vi "X509_store_get_size.vi"(8 "error in (no error)":errorcluster, 11 "SSL-Context in":refnum<class "SSL-Context.lvclass">) -> (0 "error out":errorcluster, 2 "Size of X509 Store":i32, 3 "SSL-Context out":refnum<class "SSL-Context.lvclass">)   [LabVIEW 2013, in "OpenSSL Socket.lvlib" / "SSL-Context.lvclass"]
uses:
  SSL-Context.lvclass
  SSL-Lib/SSL-Lib.lvclass/SSL-Lib.ctl
  SSL-Lib/Read Crypto Library Path.vi
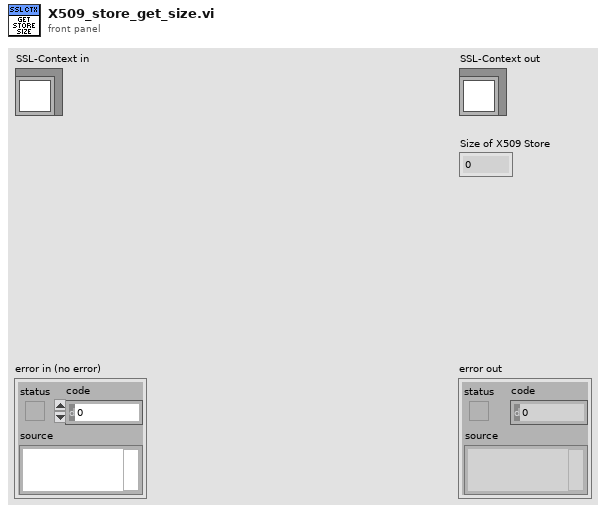
[diagram p1: front panel]
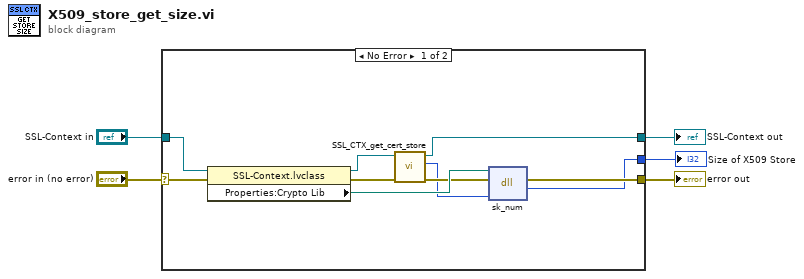
[diagram p0: block diagram]
diagram:
  n1 = case shown="No Error" "error in (no error)" {
    selector: "error in (no error)" -> [w15 w17]
    tunnel: [w12 w17] -> w4
    tunnel: [w8 w16] -> w2
    tunnel: "SSL-Context in" -> [w14 w16]
    tunnel: [w11 _] -> w1
    frame No Error {
      n2 = property class="SSL-Context.lvclass"(reference=w14, error in=w15) -> (reference out=w9:refnum<class "SSL-Context.lvclass">, error out=w10:errorcluster, "Properties:Crypto Lib"=w13:path)
      n3 = call "SSL_CTX_get_cert_store.vi"("error in (no error)"=w10, "SSL-Context in"=w9) -> ("error out"=w7:errorcluster, "X509 Cert Store"=w6:u64, "SSL-Context out"=w8:refnum<class "SSL-Context.lvclass">)  [unwired: 7 in]
      n4 = dll-call lib="C:/Program Files (x86)/National Instruments/Shared/nissl/NIlibeay32.dll" fn="sk_num"(path in=w13, error in=w7, "X509_store"=w6) -> (error out=w12:errorcluster, "return type"=w11:i32)  [unwired: 2 in, 1 out]
    }
    frame Error {
    }
  }
  "error out" <- w4
  "SSL-Context out" <- w2
  "Size of X509 Store" <- w1
